vi "Receive Page.vi"(8 "error in (no error)":errorcluster, 11 "Node Ptr":T1 format="%.0x") -> (0 "error out":errorcluster)   [LabVIEW 2023, in "Vires VTD System Explorer.lvlib"]
uses:
  Vires VTD System Explorer.lvlib
  <vilib>/NI VeriStand/Custom Device API/Custom Device Item Ref.ctl
  <vilib>/NI VeriStand/Custom Device API/Custom Device Channel.ctl
  <vilib>/NI VeriStand/Custom Device API/Custom Device Channel Type.ctl
  Shared/Constants.vi
  <vilib>/NI VeriStand/Custom Device API/Custom Device API.lvlib
  Shared/Vires VTD Shared.lvlib
  Utility/DSLV_Tree/DSLV_Tree.lvlib
panel:
  in  "no of points (if need)":u8
  in  "WheelID (if need)":u8
  in  "PlayerID":u8=1
  in  "Add to Outputs":bool
  in  "Tree":string(tree)
  in  "Header":cluster{"Section Name":string}={"Section Name"="Custom Device Item Settings"}
  in  "Description":string
  in  "Name":string
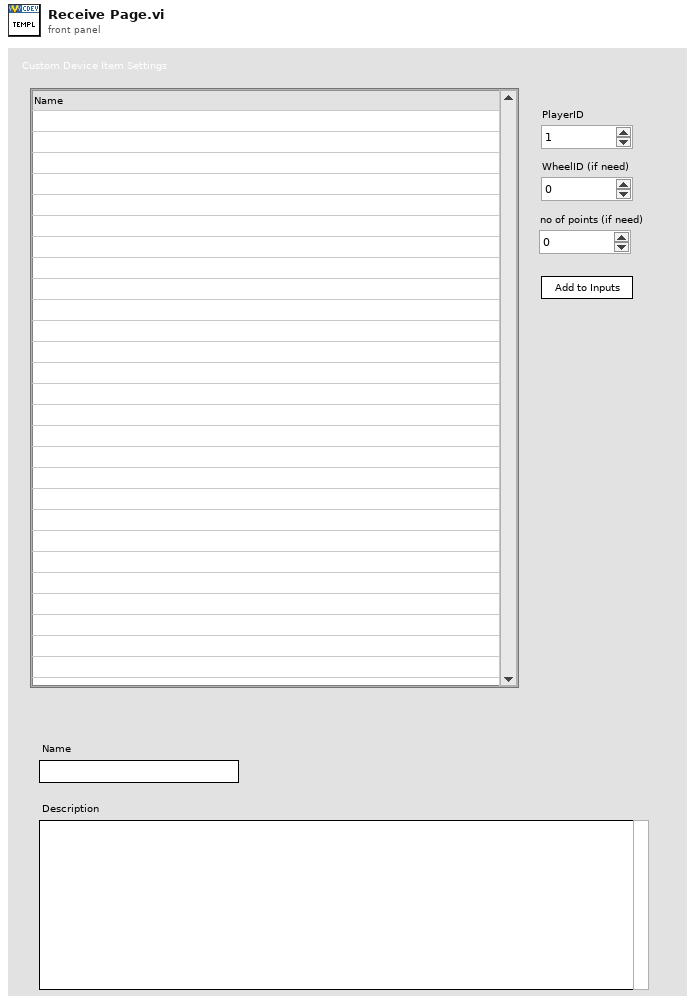
[diagram p1: front panel]
types:
  T1 = typedef "Custom Device API.lvlib/Custom Device Item Ref.ctl" = u64
  T2 = typedef "Custom Device API.lvlib/Custom Device Item Info.ctl" = cluster{"Name":string, "Is Channel":bool, "GUID":string, "Is Waveform":bool}
  T3 = cluster{"Tag":string, "Selected?":enum16{"UnSelected", "Selected", "PartSelected"}}[]
  T4 = cluster{"Tag":string, "Selected?":enum16{"UnSelected", "Selected", "PartSelected"}}
  T5 = typedef "Custom Device API.lvlib/Custom Device Channel.ctl" = cluster{"Type":T6, "Units":string, "Default Value":dbl, "Faultable":bool, "Scalable":bool}
  T6 = typedef "Custom Device API.lvlib/Custom Device Channel Type.ctl" = enum16{"Input", "Output"}
  T7 = typedef "Custom Device API.lvlib/Custom Device Commands.ctl" = enum16{"Default", "Item renamed", "Shutdown", "Dynamic button pressed"}
  T8 = typedef "LVPoint32TypeDef.ctl" = cluster{"Horizontal":i32, "Vertical":i32}
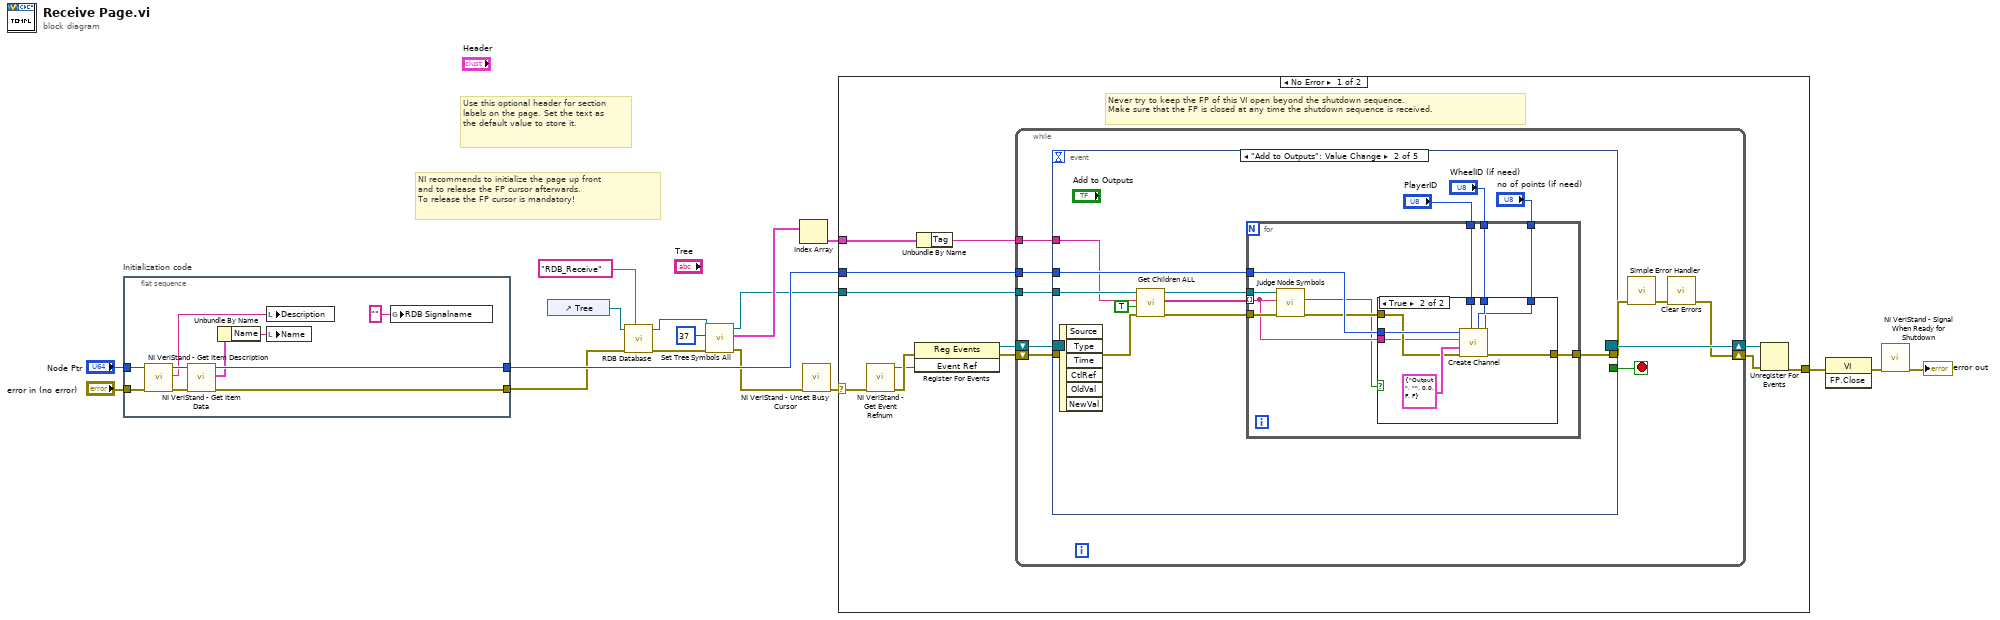
[diagram p0: block diagram]
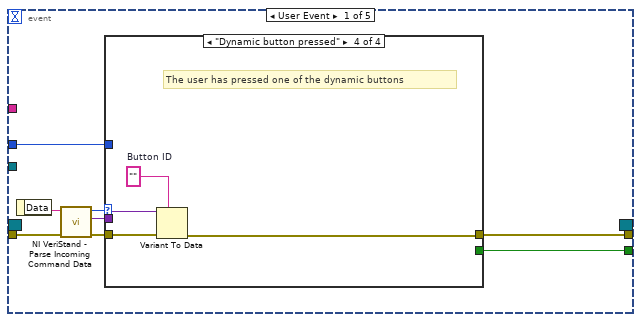
[diagram p2: hidden frame]
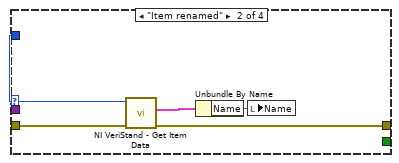
[diagram p4: hidden frame]
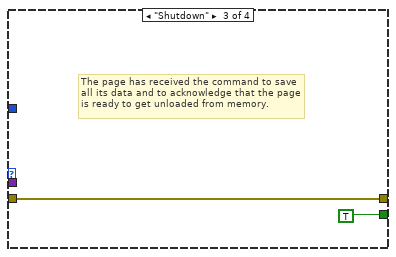
[diagram p5: hidden frame]
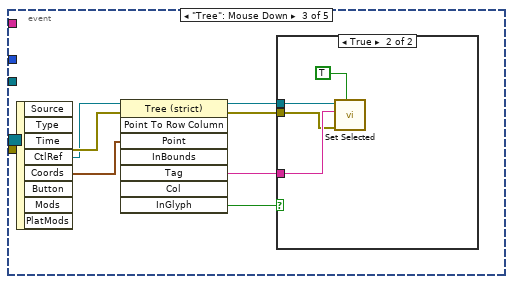
[diagram p7: hidden frame]
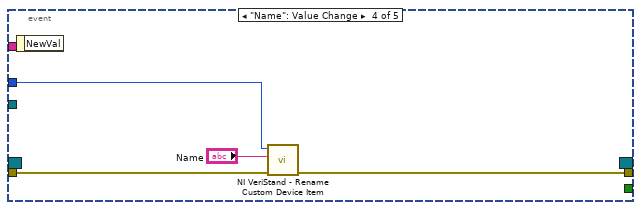
[diagram p9: hidden frame]
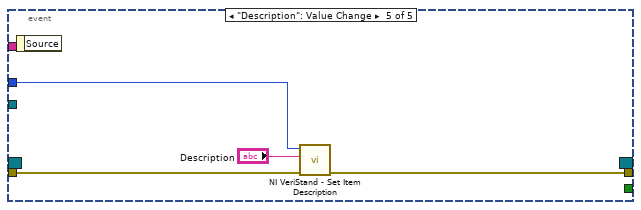
[diagram p10: hidden frame]
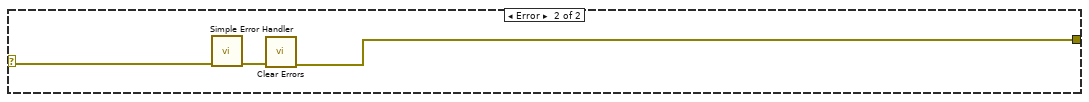
[diagram p11: hidden frame]
diagram:
  # "Use this optional header for section labels on the page. Set the text as the default value to store it."
  # "NI recommends to initialize the page up front\nand to release the FP cursor afterwards.\nTo release the FP cursor is mandatory!"
  n1 = flat-sequence "Initialization code" {
    tunnel: "error in (no error)" -> [w25]
    tunnel: "Node Ptr" -> [w24]
    tunnel: [w19] -> w10
    tunnel: [w27] -> w11
    frame #0 {
      n2 = call <vilib>:"NI VeriStand - Get Item Description.vi"("error in (no error)"=w25, "Item Ref in"=w24) -> ("error out"=w22:errorcluster, "Description"=w23:string, "Item Ref out"=w26:T1)  [unwired: 7 out]
      n3 = call <vilib>:"NI VeriStand - Get Item Data.vi"("error in (no error)"=w22, "Item Ref in"=w26) -> ("error out"=w19:errorcluster, "Item Info"=w21:T2, "Item Ref out"=w27:T1)  [unwired: 7 out]
      n4 = Unbundle By Name(w21) -> ("Name"=w20:string)
      n5 = local write "Description"(w23) -> ()
      n6 = local write "Name"(w20) -> ()
      n7 = global write "Constants.vi" "RDB Signalname"("" ("RDB Signalname")) -> ()
    }
  }
  n8 = control-ref of="Tree"() -> (w9:refnum<vi>)
  n9 = call "RDB Database.vi"("Filter Cluster"="RDB_Receive", "error in (no error)"=w10, "reference in"=w9) -> ("error out"=w6:errorcluster, "reference out"=w4:refnum<vi>)  [unwired: 7 in]
  n10 = call "Set Tree Symbols All.vi"("error in (no error)"=w6, "symbol"=37, "Tree Refnum"=w4) -> ("error out"=w5:errorcluster, "Seted Tags"=w3:T3, "Tree Refnum"=w1:refnum<vi>)  [unwired: 6 in]
  n11 = Index Array(array=w3) -> (element=w2:T4)  [unwired: 1 in]
  n12 = call <vilib>:"NI VeriStand - Unset Busy Cursor.vi"("error in (no error)"=w5) -> ("error out"=w13:errorcluster)  [unwired: 10 out]
  n13 = case shown="No Error" w13 {
    selector: w13 -> [w31 w122]
    tunnel: [w36 w120] -> w17
    tunnel: w11 -> [w32 _]
    tunnel: w2 -> [w30 _]
    tunnel: w1 -> [w29 _]
    frame No Error {
      # "Never try to keep the FP of this VI open beyond the shutdown sequence.\nMake sure that the FP is closed at any time the shutdown sequence is received."
      n14 = call <vilib>:"NI VeriStand - Get Event Refnum.vi"("error in (no error)"=w31) -> ("error out"=w39:errorcluster, "Event Ref"=w35:refnum<user-event>)  [unwired: 9 out]
      n15 = register-events(error in=w39, w35) -> (reference out=w33:refnum<event-registration>, error out=w34:errorcluster)  [unwired: 1 in]
      n16 = Unbundle By Name(w30) -> ("Tag"=w28:string)
      n17 = while {
        tunnel: w32 -> [w45]
        shift-right: [w42] -> w37
        shift-left: w34 -> [w48]
        shift-right: [w49] -> w38
        shift-left: w33 -> [w47]
        tunnel: w29 -> [w41]
        tunnel: w28 -> [w40]
        stop <- w46 stop-if-true
        n18 = event shown="[1] \"Add to Outputs\": Value Change" {
          selector: w47 -> [_ _ _ _ _]
          dyn-events: [_ _ _ _ _] -> w49
          timeout: _ -> [_ _ _ _ _]
          tunnel: w48 -> [w57 w75 w107 w115 w118]
          tunnel: [w53 _ _ _ _] -> w46
          tunnel: [w52 w80 _ w114 w117] -> w44
          tunnel: w45 -> [w51 w81 _ w113 w119]
          tunnel: w41 -> [_ w78 _ _ _]
          tunnel: w40 -> [_ w77 _ _ _]
          event User Event {
            n19 = event-data() -> ("Data"=w56:string)  [unwired: 1 out]
            n20 = call <vilib>:"NI VeriStand - Parse Incoming Command Data.vi"("error in (no error)"=w57, "Incoming data"=w56) -> ("error out"=w55:errorcluster, "Outgoing data"=w50:variant, "Action"=w54:T7)  [unwired: 7 out]
            n21 = case shown="\"Dynamic button pressed\"" w54 {
              tunnel: w55 -> [w58 w63 w64 w69]
              tunnel: [_ _ TRUE _] -> w53
              tunnel: [w58 w60 w64 w66] -> w52
              tunnel: w51 -> [_ w62 _ _]
              tunnel: w50 -> [_ _ _ w68]
              frame "Default", Default {
              }
              frame "Item renamed" {
                n22 = call <vilib>:"NI VeriStand - Get Item Data.vi"("error in (no error)"=w63, "Item Ref in"=w62) -> ("error out"=w60:errorcluster, "Item Info"=w61:T2)  [unwired: 8 out]
                n23 = Unbundle By Name(w61) -> ("Name"=w59:string)
                n24 = local write "Name"(w59) -> ()
              }
              frame "Shutdown" {
                # "The page has received the command to save all its data and to acknowledge that the page is ready to get unloaded from memory."
              }
              frame "Dynamic button pressed" {
                w67 = ""  # Button ID
                # "The user has pressed one of the dynamic buttons"
                n25 = Variant To Data(error in=w69, type=w67, Variant=w68) -> (error out=w66:errorcluster)  [unwired: 1 out]
              }
            }
          }
          event "Add to Outputs": Value Change {
            n26 = event-data() -> ()  [unwired: 7 out]
            n27 = call "Get Children ALL.vi"("error in"=w75, "pure children？"=TRUE, "Parent Tag"=w77, "Tree Reference"=w78) -> ("error out"=w72:errorcluster, "Children Tags"=w74:string[], "Tree Reference"=w73:refnum<vi>)  [unwired: 5 in]
            n28 = for {
              tunnel: w81 -> [w91]
              tunnel: [w90] -> w80
              tunnel: "PlayerID" -> [w89]
              tunnel: w74 -> [w86] mode=indexing
              tunnel: w73 -> [w88]
              tunnel: w72 -> [w87]
              tunnel: "WheelID (if need)" -> [w83]
              tunnel: "no of points (if need)" -> [w82]
              n29 = call "Judge Node Symbols.vi"("error in (no error)"=w87, "Tag"=w86, "TreeControl in"=w88) -> ("error out"=w85:errorcluster, "Selected?"=w84:bool)  [unwired: 6 in, 1 out]
              n30 = case shown="True" w84 {
                tunnel: w91 -> [_ w100]
                tunnel: [w92 w99] -> w90
                tunnel: w89 -> [_ w98]
                tunnel: w86 -> [_ w95]
                tunnel: w85 -> [w92 w96]
                tunnel: w83 -> [_ w94]
                tunnel: w82 -> [_ w93]
                frame False {
                }
                frame True {
                  n31 = call "Create Channel.vi"("no of points"=w93, "WheelID (if need)"=w94, "PlayerID"=w98, "error in (no error)"=w96, "Channel"=T5 {"Type"=enum."Output", "Units"="", "Default Value"=0.0, "Faultable"=FALSE, "Scalable"=FALSE}, "RDB Signalname"=w95, "Item Ref in"=w100) -> ("error out"=w99:errorcluster)  [unwired: 4 in]
                }
              }
            }
          }
          event "Tree": Mouse Down {
            n32 = event-data() -> ("CtlRef"=w106:refnum<vi>, "Coords"=w105:T8)  [unwired: 7 out]
            n33 = invoke on="Invoke Node" class="Tree (strict)" method="Point To Row Column"(reference=w106, error in=w107, "Point"=w105) -> (reference out=w102:refnum<vi>, error out=w101:errorcluster, "Tag"=w103:string, "InGlyph"=w104:bool)  [unwired: 5 in, 4 out]
            n34 = case shown="True" w104 {
              tunnel: w103 -> [_ w109]
              tunnel: w102 -> [_ w110]
              tunnel: w101 -> [_ w108]
              frame False {
              }
              frame True {
                n35 = call "Set Selected.vi"("Tri-State?"=TRUE, "error in (no error)"=w108, "Tag"=w109, "Tree Reference"=w110) -> ()  [unwired: 5 in, 3 out]
              }
            }
          }
          event "Name": Value Change {
            n36 = event-data() -> ()  [unwired: 2 out]
            n37 = call <vilib>:"NI VeriStand - Rename Custom Device Item.vi"("error in (no error)"=w115, "New Name"="Name", "Item Ref in"=w113) -> ("error out"=w114:errorcluster)  [unwired: 1 in, 7 out]
          }
          event "Description": Value Change {
            n38 = event-data() -> ()  [unwired: 2 out]
            n39 = call <vilib>:"NI VeriStand - Set Item Description.vi"("error in (no error)"=w118, "Description"="Description", "Item Ref in"=w119) -> ("error out"=w117:errorcluster)  [unwired: 8 out]
          }
        }
        n40 = call <vilib>:"Simple Error Handler.vi"("error in (no error)"=w44) -> ("error out"=w43:errorcluster)  [unwired: 1 in, 7 out]
        n41 = call <vilib>:"Clear Errors.vi"("error in (no error)"=w43) -> ("error out"=w42:errorcluster)  [unwired: 1 in, 5 out]
      }
      n42 = Unregister For Events(event registration refnum=w38, error in=w37) -> (error out=w36:errorcluster)
    }
    frame Error {
      n43 = call <vilib>:"Simple Error Handler.vi"("error in (no error)"=w122) -> ("error out"=w121:errorcluster)  [unwired: 1 in, 7 out]
      n44 = call <vilib>:"Clear Errors.vi"("error in (no error)"=w121) -> ("error out"=w120:errorcluster)  [unwired: 1 in, 5 out]
    }
  }
  n45 = invoke class="VI" method="FP.Close"(error in=w17) -> (error out=w16:errorcluster)  [unwired: 2 in, 2 out]
  n46 = call <vilib>:"NI VeriStand - Signal When Ready for Shutdown.vi"("error in (no error)"=w16) -> ("error out"=→"error out":errorcluster)  [unwired: 10 out]
